vi "Tools Pallete.vi"() -> ()   [LabVIEW 2021]
panel:
  in  "?":bool
  out "LED":bool
  in  "Toggle":bool
  out "Thermometer":dbl(slide) scale=0.0..100.0
  in  "Slide":dbl(slide) scale=0.0..100.0
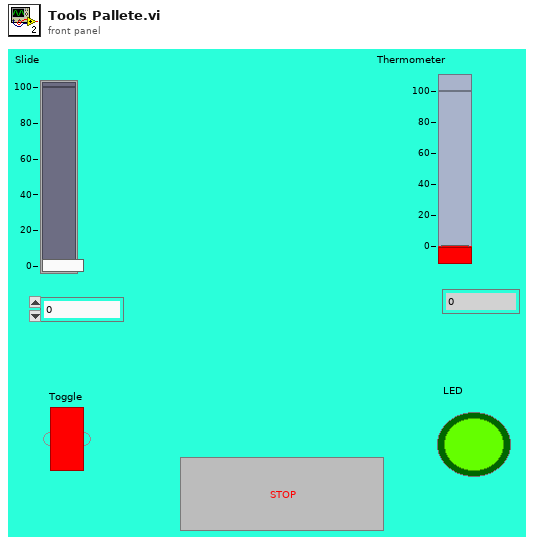
[diagram p1: front panel]
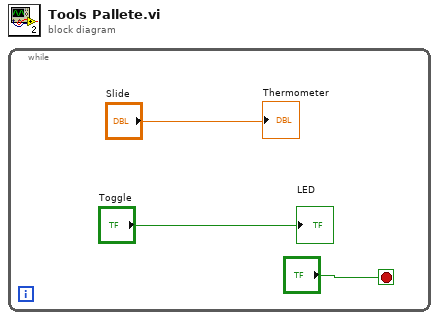
[diagram p0: block diagram]
diagram:
  n1 = while {
    stop <- "?" stop-if-true
    "Thermometer" <- "Slide"
    "LED" <- "Toggle"
  }
